vi "Bind to Type - Serializable Class - Returns Same Type.vi"() -> ()   [LabVIEW 2017, in "JSON Serializable Binder Tests.lvlib"]
uses:
  JSON Serializable Binder Tests.lvlib
  Fake JSON Serializable/Fake JSON Serializable.lvclass
  JSON Serializable Binder/JSON Serializable Binder.lvclass
  <vilib>/addons/_JKI Toolkits/Caraya/classes/Assert/Assert Equal Value and Type_Variant.vi
  <vilib>/addons/_JKI Toolkits/Caraya/classes/Test/Test.lvclass
  <vilib>/addons/_JKI Toolkits/Caraya/classes/Assert/Assert.lvclass
panel:
  out "error out":errorcluster
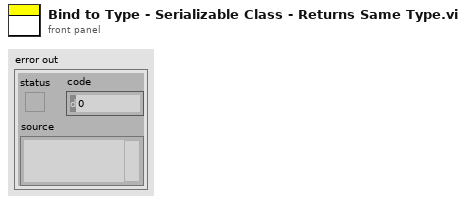
[diagram p1: front panel]
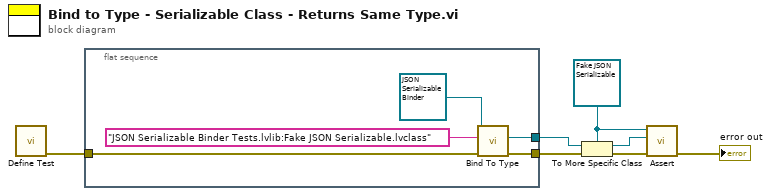
[diagram p0: block diagram]
diagram:
  w1 = refnum<class "Fake JSON Serializable.lvclass"> refnum ("target class")
  n1 = call <vilib>:"Define Test.vi"() -> ("error out"=w6:errorcluster)  [unwired: 11 in]
  n2 = flat-sequence {
    tunnel: w6 -> [w12]
    tunnel: [w9] -> w3
    tunnel: [w8] -> w2
    frame #0 {
      n3 = call-dynamic "Bind To Type.vi"("error in (no error)"=w12, "Type Name"="JSON Serializable Binder Tests.lvlib:Fake JSON Serializable.lvclass", "JSON Serializable Binder in"=refnum<class "JSON Serializable Binder.lvclass"> refnum ("JSON Serializable Binder.lvclass")) -> ("error out"=w9:errorcluster, "Type"=w8:refnum<class>)  [unwired: 6 in, 1 out]
    }
  }
  n4 = To More Specific Class(target class=w1, reference=w2, error in=w3) -> (specific class reference=w4:refnum<class "Fake JSON Serializable.lvclass">, error out=w7:errorcluster)
  n5 = call-poly <vilib>:"Assert.vi"("error in (no error)"=w7, "Y"=w4, "X"=w1) -> ("error out"=→"error out":errorcluster)  [unwired: 8 in]
